vi "Write Core.vi"(8 "error in (no error)":errorcluster, 10 "PV":refnum<class "PV.lvclass">, 11 "DIMConnection in":refnum<class "DIMConnection.lvclass">) -> (0 "error out":errorcluster, 3 "DIMConnection out":refnum<class "DIMConnection.lvclass">)   [LabVIEW 2014, in "CS++DIM.lvlib" / "DIMConnection.lvclass"]
doc: "Publish a process varibale."
uses:
  DIMConnection.lvclass
  DimLVEvent/LVDimInterface/LVDimInterface.lvlib
  CSPP_Core/Classes/CS++ProcessVariables/ProcessVariable/PV.lvclass
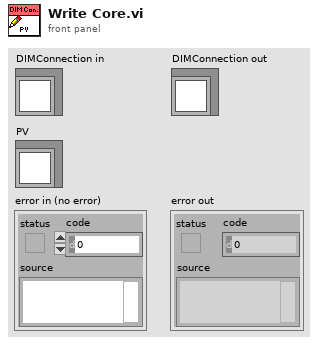
[diagram p1: front panel]
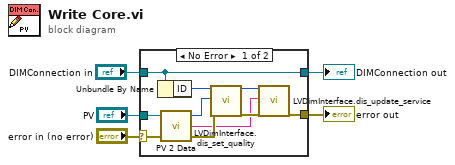
[diagram p0: block diagram]
diagram:
  n1 = case shown="No Error" "error in (no error)" {
    selector: "error in (no error)" -> [w9 w16]
    tunnel: "PV" -> [w10 _]
    tunnel: "DIMConnection in" -> [w11 w17]
    tunnel: [w12 w16] -> w3
    tunnel: [w11 w17] -> w1
    frame No Error {
      n2 = Unbundle By Name(w11) -> ("ID"=w15:i32)
      n3 = call "PV 2 Data.vi"("Error In"=w9, "PV"=w10) -> ("Error Out"=w7:errorcluster, "Data"=w6:string, "Quality"=w8:i32)  [unwired: 1 in]
      n4 = call "LVDimInterface.dis_set_quality.vi"("my_serviceID"=w15, "quality"=w8, "error in (no error)"=w7) -> ("my_serviceID (out)"=w14:i32, "error out"=w13:errorcluster)  [unwired: 15 in]
      n5 = call "LVDimInterface.dis_update_service.vi"("my_serviceID"=w14, "data"=w6, "error in (no error)"=w13) -> ("error out"=w12:errorcluster)  [unwired: 14 in, 2 out]
    }
    frame Error {
    }
  }
  "error out" <- w3
  "DIMConnection out" <- w1
